vi "Read External Start.vi"(8 "error in (no error)":errorcluster, 11 "JQMHModule in":refnum<class "Module.lvclass">) -> (0 "error out":errorcluster, 2 "External Start?":bool, 3 "JQMHModule out":refnum<class "Module.lvclass">)   [LabVIEW 2024, in "Module.lvclass"]
uses:
  Module.lvclass
  Module.lvclass/Module.ctl
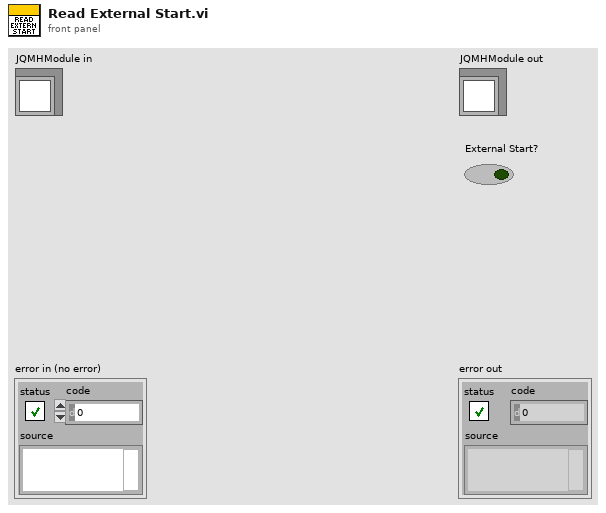
[diagram p1: front panel]
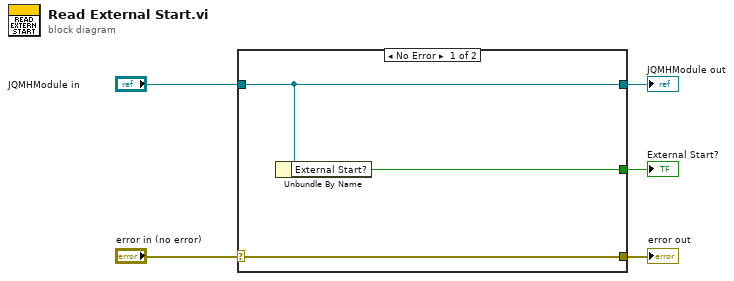
[diagram p0: block diagram]
diagram:
  n1 = case shown="No Error" "error in (no error)" {
    selector: "error in (no error)" -> [w8 w9]
    tunnel: [w8 w9] -> w4
    tunnel: [w7 w10] -> w2
    tunnel: "JQMHModule in" -> [w7 w10]
    tunnel: [w6 _] -> w1
    frame No Error {
      n2 = Unbundle By Name(w7) -> ("External Start?"=w6:bool)
    }
    frame Error {
    }
  }
  "error out" <- w4
  "JQMHModule out" <- w2
  "External Start?" <- w1
